vi "Start Recipe.vi"(8 "error in (no error)":errorcluster, 10 "Recipe File":path, 11 "Recipe Controller in":refnum<class "Recipe Controller.lvclass">) -> (0 "error out":errorcluster, 3 "Recipe Controller out":refnum<class "Recipe Controller.lvclass">)   [LabVIEW 2022 SP3, in "Recipe Controller.lvclass"]
uses:
  Recipe Controller.lvclass
  Recipe Controller.lvclass/Recipe Controller.ctl
  Recipe Process/Recipe Process Messages/Start Recipe Msg/Start Recipe Msg.lvclass/Start Recipe Msg.ctl
  Recipe Process/Recipe Process Messages/Start Recipe Msg/Start Recipe Msg.lvclass
  C:/Program Files/National Instruments/LabVIEW 2022/vi.lib/ActorFramework/Message/Message.lvclass
  XY Stage/Process Actor/Process Framework/Interlock Q Class/Interlock Q Class.lvclass
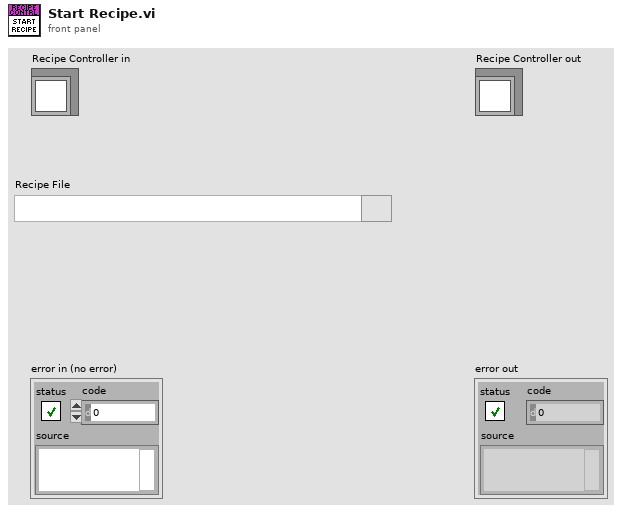
[diagram p1: front panel]
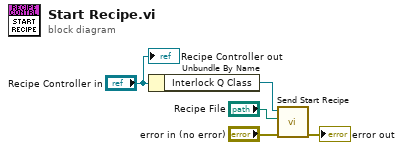
[diagram p0: block diagram]
diagram:
  n1 = Unbundle By Name("Recipe Controller in") -> ("Interlock Q Class"=w3:refnum<class "Interlock Q Class.lvclass">)
  n2 = call "Send Start Recipe.vi"("error in (no error)"="error in (no error)", "Recipe File"="Recipe File", "Interlock Q Class"=w3) -> ("error out"=→"error out":errorcluster)  [unwired: 7 in, 1 out]
  "Recipe Controller out" <- "Recipe Controller in"
